vi "CONEX-ALL Get Identifier v2.vi"(11 "Connection Cluster in":T1) -> (1 "Identifier":string, 3 "Connection Cluster out":T1)   [LabVIEW 2013]
doc: "ID? - Get Identifier\n\nIdentifier is for attached device. (e.g. optical sensor, motion stage, etc.)\n\nReturn: Identifier string"
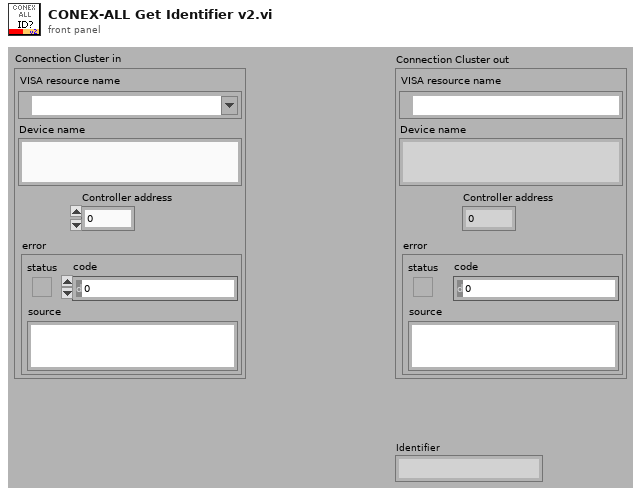
[diagram p1: front panel]
types:
  T1 = cluster{"VISA resource name":refnum<visa-resource-name>, "Device name":string, "Controller address":i32, "error":errorcluster}
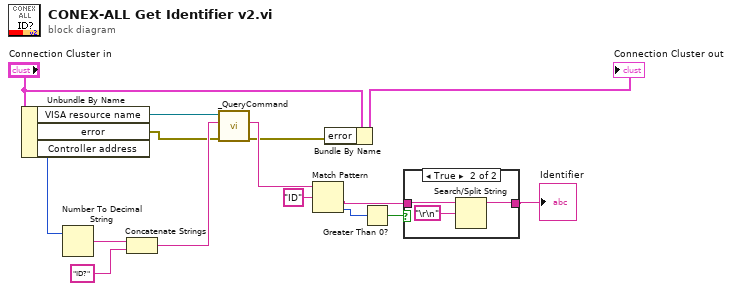
[diagram p0: block diagram]
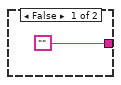
[diagram p2: hidden frame]
diagram:
  n1 = Unbundle By Name("Connection Cluster in") -> ("VISA resource name"=w8:refnum<visa-resource-name>, "error"=w6:errorcluster, "Controller address"=w1:i32)
  n2 = Number To Decimal String(number=w1) -> (decimal integer string=w15:string)  [unwired: 1 out]
  n3 = Concatenate Strings(w15, "ID?" ("strCommand")) -> (w7:string)
  n4 = call "_QueryCommand.vi"("error in"=w6, "Command"=w7, "Instrument Channel in"=w8) -> ("error out"=w3:errorcluster, "Response"=w5:string)  [unwired: 6 in, 1 out]
  n5 = Match Pattern(string=w5, regular expression="ID" ("expression régulière")) -> (after substring=w12:string, offset past match=w11:i32)  [unwired: 3 out]
  n6 = Bundle By Name(cluster="Connection Cluster in", "error"=w3) -> (→"Connection Cluster out":T1)
  n7 = Greater Than 0?(x=w11) -> (x > 0?=w10:bool)
  n8 = case shown="True" w10 {
    tunnel: w12 -> [_ w18]
    tunnel: ["" w17] -> w9
    frame False {
    }
    frame True {
      n9 = Search/Split String(string=w18, search string/char (-)="\r\n") -> (substring before match=w17:string)  [unwired: 3 out]
    }
  }
  "Identifier" <- w9
